vi "Ultrasonic Update.vi"(11 "SonarMB1010AnalogDevRef":T1={"AIDeviceRef"={"DevStatus"={"status"=FALSE, "code"=0, "source"=""}, "Analog Channel"=enum."Invalid"}, "Scaling factor (V/in)"=0.0098, "Average Bits"=3} {"Average Bits" max=15}) -> (3 "SonarMB1010AnalogDevRef 2":T1={"AIDeviceRef"={"DevStatus"={"status"=FALSE, "code"=0, "source"=""}, "Analog Channel"=enum."Invalid"}, "Scaling factor (V/in)"=0.0098, "Average Bits"=3} {"Average Bits" max=15})   [LabVIEW 2015]
uses:
  <vilib>/Rock Robotics/WPI/Ultrasonic/WPI_SonarMB1010AnalogDeviceRef.ctl
  <vilib>/Rock Robotics/WPI/AnalogChannel/WPI_AnalogChannelDevRef.ctl
  <vilib>/Rock Robotics/SystemInterfaces/AI/FPGA_AIChannel.ctl
  <vilib>/Rock Robotics/WPI/Ultrasonic/WPI_SonarMB1010AnalogGetRange.vi
  <vilib>/Rock Robotics/Network Tables/NT Write Number.vi
  Robot Values.vi
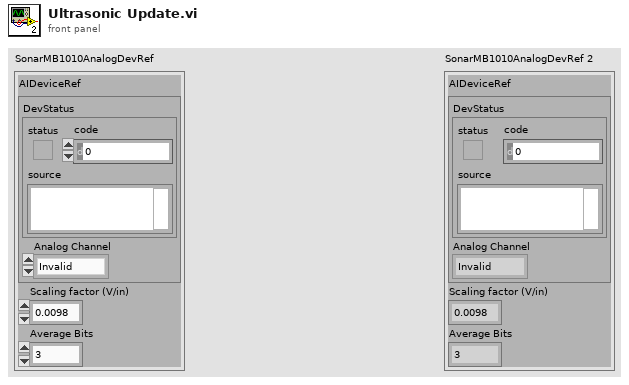
[diagram p1: front panel]
types:
  T1 = typedef "WPI_SonarMB1010AnalogDeviceRef.ctl" = cluster{"AIDeviceRef":T2, "Scaling factor (V/in)":dbl, "Average Bits":u8}
  T2 = typedef "WPI_AnalogChannelDevRef.ctl" = cluster{"DevStatus":errorcluster, "Analog Channel":T3}
  T3 = typedef "FPGA_AIChannel.ctl" = enum8{"AI 0", "AI 1", "AI 2", "AI 3", "AI MXP 0", "AI MXP 1", "AI MXP 2", "AI MXP 3", "Invalid"}
  T4 = typedef "Drive Values.ctl" = cluster{"Drive Motors":cluster{"Left Motor Value":dbl, "Right Motor Value":dbl}, "Sensors":cluster{"Gyro Angle":dbl, "Ultrasonic Range":dbl}}
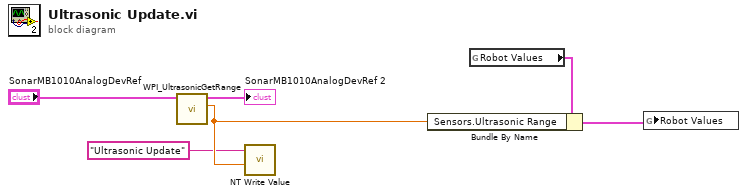
[diagram p0: block diagram]
diagram:
  n1 = call-poly <vilib>:"WPI_UltrasonicGetRange.vi"("SonarMB1010AnalogDevRef"="SonarMB1010AnalogDevRef") -> ("Distance"=w4:dbl, "SonarMB1010AnalogDevRef"=→"SonarMB1010AnalogDevRef 2":T1)  [unwired: 8 in, 1 out]
  n2 = call-poly <vilib>:"NT Write Value.vi"("Numeric"=w4, "Name"="Ultrasonic Update") -> ()  [unwired: 9 in, 1 out]
  n3 = global read "Robot Values.vi" "Robot Values"() -> (w3:T4)
  n4 = Bundle By Name(cluster=w3, "Sensors.Ultrasonic Range"=w4) -> (w2:T4)
  n5 = global write "Robot Values.vi" "Robot Values"(w2) -> ()
